vi "conversionConfigU8.vi"(1 "Config":T1={"action"=enum."PIV", "nb_periodes"=0, "t_periode"=1, "nb_pulse_prechauffe"=0, "nb_skip_frame_PIV"=0, "nb_skip_frame_LAT"=0, "t_FL1_start"=0, "t_FL1_stop"=0, "t_QS1_start"=0, "t_QS1_stop"=0, "t_FL2_start"=0, "t_FL2_stop"=0, "t_QS2_start"=0, "t_QS2_stop"=0, "t_LAT_start"=0, "t_LAT_stop"=0, "t_FRAME1_start"=0, "t_FRAME1_stop"=0, "t_FRAME2_start"=0, "t_FRAME2_stop"=0}) -> (0 "TrameConsigne":string)   [LabVIEW 2023]
uses:
  configFPGA.ctl
  convU16[U8].vi
  convU32[U8].vi
panel:
  out "size(s)":i32
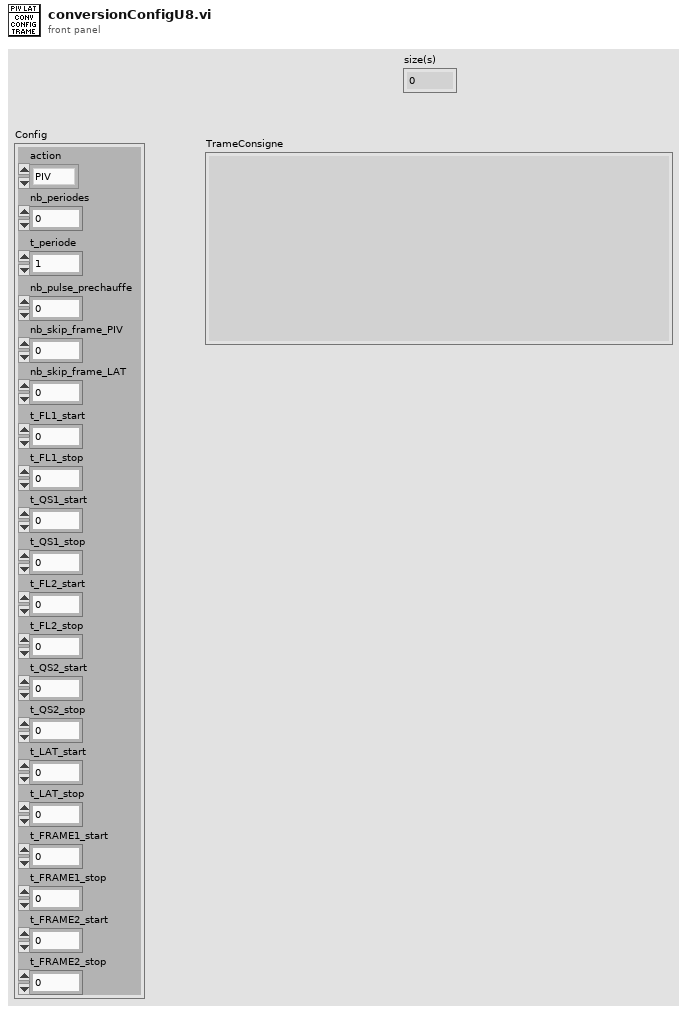
[diagram p1: front panel]
types:
  T1 = typedef "configFPGA.ctl" = cluster{"action":enum8{"PIV", "PIV + LAT", "LAT", "STOP"}, "nb_periodes":u16, "t_periode":u32, "nb_pulse_prechauffe":u8, "nb_skip_frame_PIV":u8, "nb_skip_frame_LAT":u8, "t_FL1_start":u32, "t_FL1_stop":u32, "t_QS1_start":u32, "t_QS1_stop":u32, "t_FL2_start":u32, "t_FL2_stop":u32, "t_QS2_start":u32, "t_QS2_stop":u32, "t_LAT_start":u32, "t_LAT_stop":u32, "t_FRAME1_start":u32, "t_FRAME1_stop":u32, "t_FRAME2_start":u32, "t_FRAME2_stop":u32}
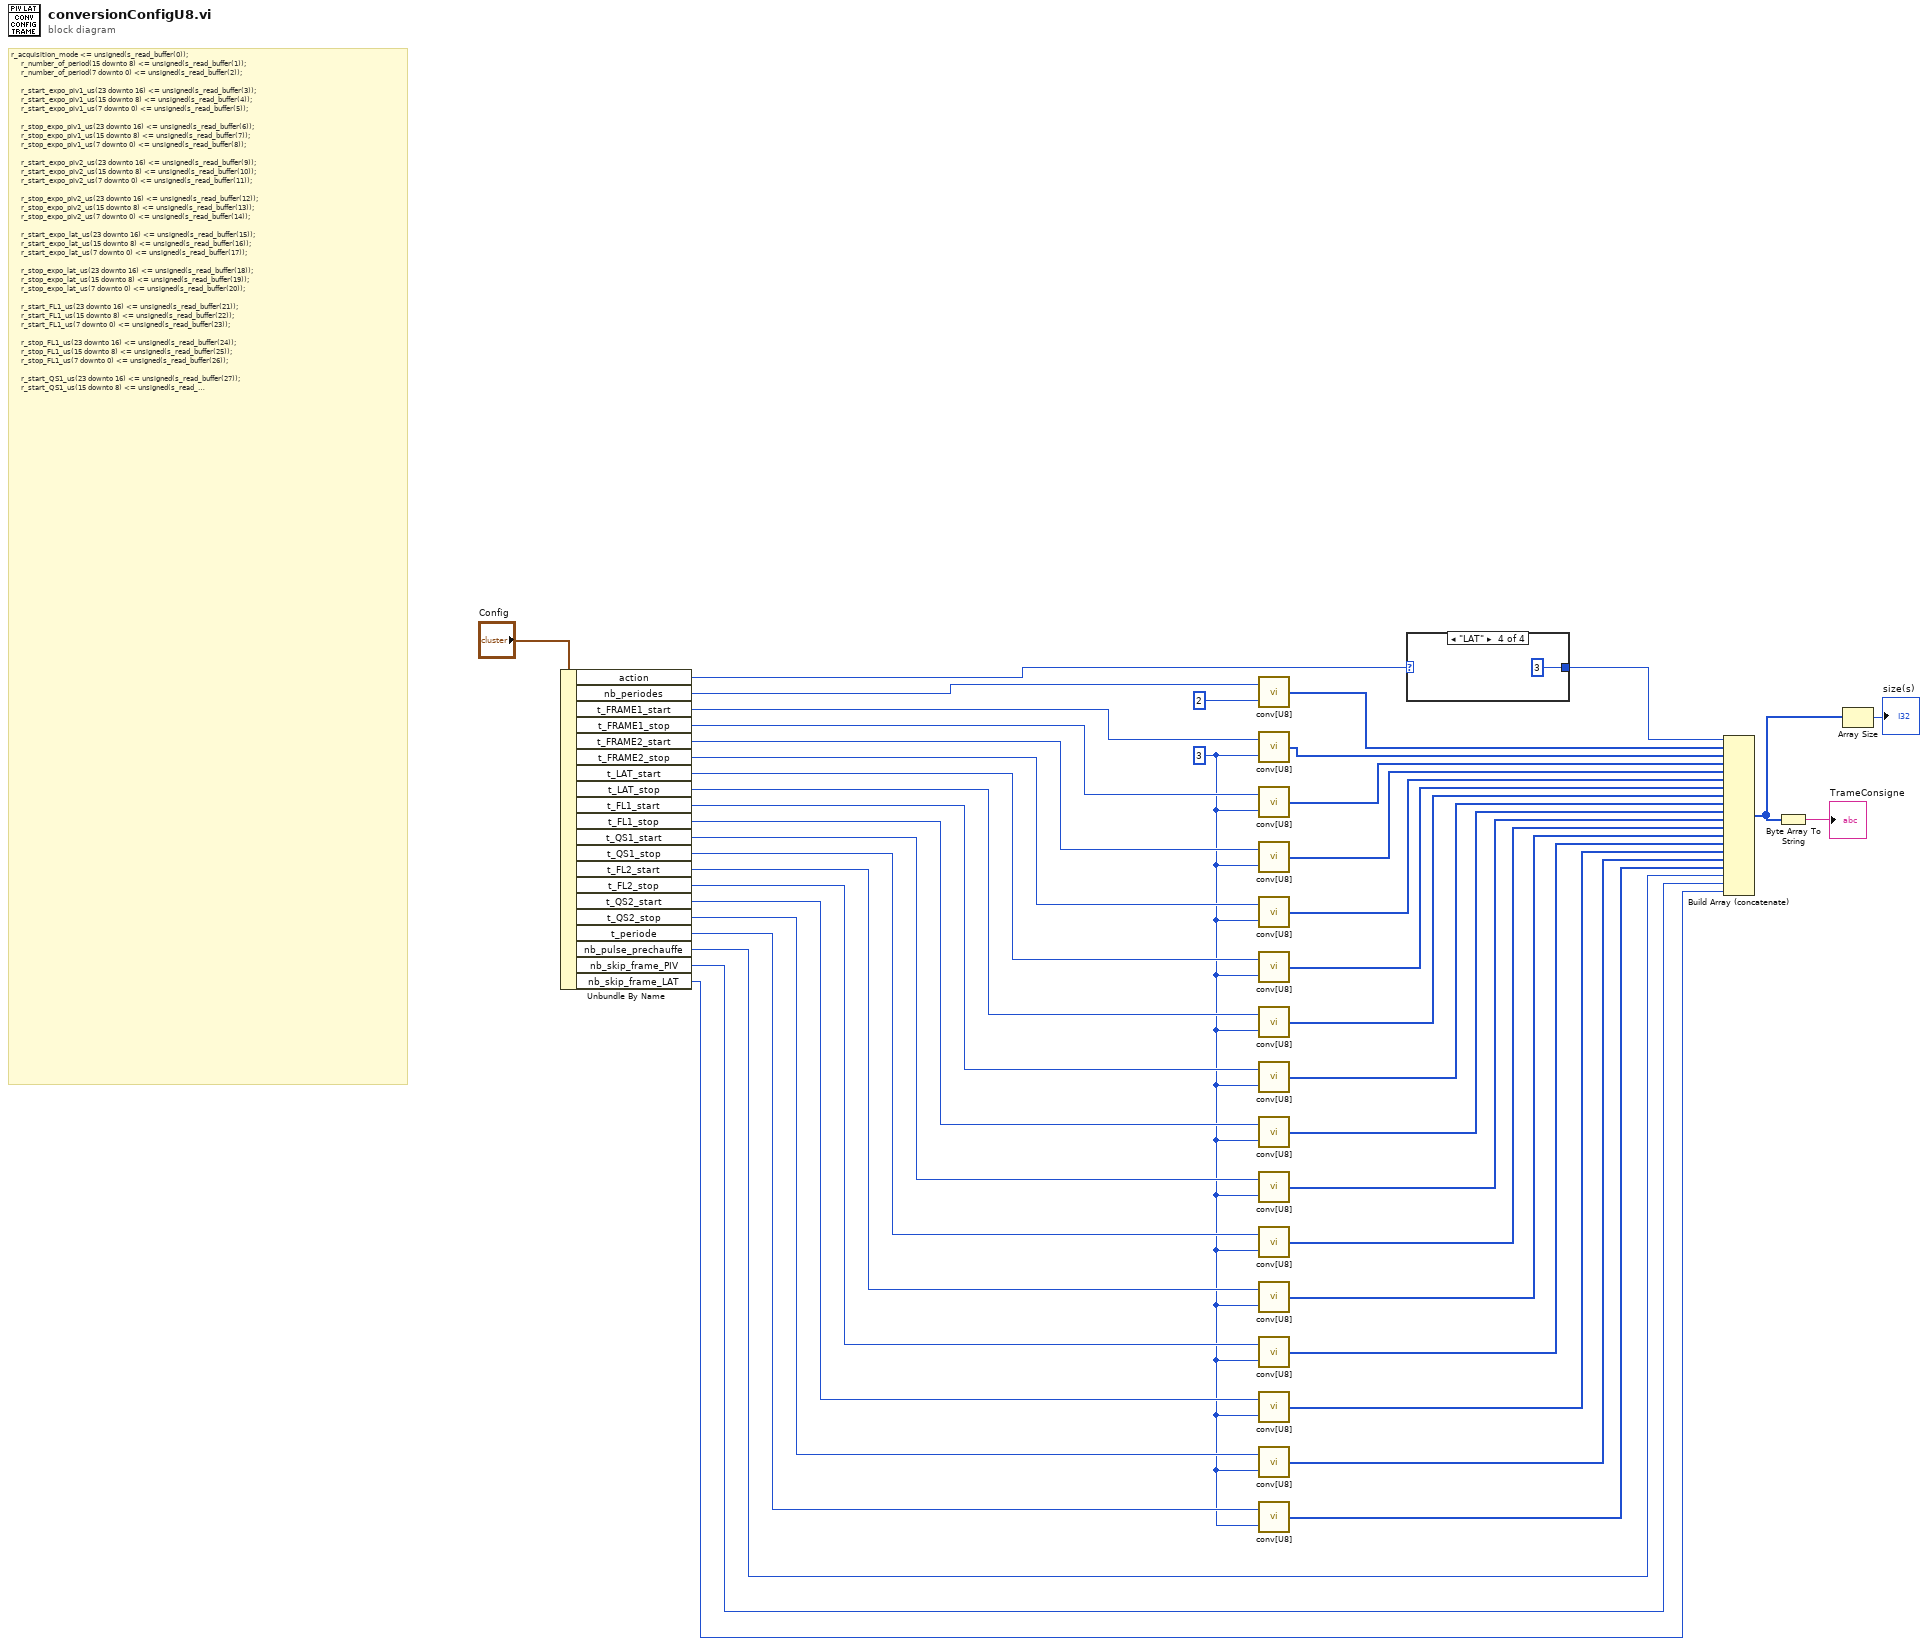
[diagram p0: block diagram]
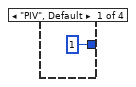
[diagram p2: hidden frame]
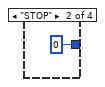
[diagram p3: hidden frame]
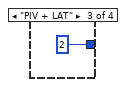
[diagram p4: hidden frame]
diagram:
  w17 = 3 ("dimension size")
  # "r_acquisition_mode <= unsigned(s_read_buffer(0));\n     r_number_of_period(15 downto 8) <= unsigned(s_read_buffer(1));\n\t\t\t\t\tr_number_of_period(7 downto 0) <= unsigned(s_read_buffer(2));\n\t\t\t\t\t\n\t\t\t\t\tr_start_expo_piv1_us(23 downto 16) <= unsigned(s_read_buffer(3));\n\t\t\t\t\tr_start_expo_piv1_us(15 downto 8) <= unsigned(s_read_buffer(4));\n\t\t\t\t\tr_start_expo_piv1_us(7 downto 0) <= unsigned(s_read_buffer(5));\n\t\t\t\t\t\n\t\t\t\t\tr_stop_expo_piv1_us(23 downto 16) <= unsigned(s_read_buffer(6));\n\t\t\t\t\tr_stop_expo_piv1_us(15 downto 8) <= unsigned(s_read_buffer(7));\n\t\t\t\t\tr_stop_expo_piv1_us(7 downto 0) <= unsigned(s_read_buffer(8));\n\t\t\t\t\t\n\t\t\t\t\tr_start_expo_piv2_us(23 downto 16) <= unsigned(s_read_buffer(9));\n\t\t\t\t\tr_start_expo_piv2_us(15 downto 8) <= unsigned(s_read_buffer(10));\n\t\t\t\t\tr_start_expo_piv2_us(7 downto 0) <= unsigned(s_read_buffer(11));\n\t\t\t\t\t\n\t\t\t\t\tr_stop_expo_piv2_us(23 downto 16) <= unsigned(s_read_buffer(12));\n\t\t\t\t\tr_stop_expo_piv2_us(15 downto 8) <= unsigned(s_read_buffer(13));\n\t\t\t\t\tr_stop_expo_piv2_us(7 downto 0) <= unsigned(s_read_buffer(14));\n\t\t\t\t\t\n\t\t\t\t\tr_start_expo_lat_us(23 downto 16) <= unsigned(s_read_buffer(15));\n\t\t\t\t\tr_start_expo_lat_us(15 downto 8) <= unsigned(s_read_buffer(16));\n\t\t\t\t\tr_start_expo_lat_us(7 downto 0) <= unsigned(s_read_buffer(17));\n\t\t\t\t\t\n\t\t\t\t\tr_stop_expo_lat_us(23 downto 16) <= unsigned(s_read_buffer(18));\n\t\t\t\t\tr_stop_expo_lat_us(15 downto 8) <= unsigned(s_read_buffer(19));\n\t\t\t\t\tr_stop_expo_lat_us(7 downto 0) <= unsigned(s_read_buffer(20));\n\t\t\t\t\t\n\t\t\t\t\tr_start_FL1_us(23 downto 16) <= unsigned(s_read_buffer(21));\n\t\t\t\t\tr_start_FL1_us(15 downto 8) <= unsigned(s_read_buffer(22));\n\t\t\t\t\tr_start_FL1_us(7 downto 0) <= unsigned(s_read_buffer(23));\n\t\t\t\t\t\n\t\t\t\t\tr_stop_FL1_us(23 downto 16) <= unsigned(s_read_buffer(24));\n\t\t\t\t\tr_stop_FL1_us(15 downto 8) <= unsigned(s_read_buffer(25));\n\t\t\t\t\tr_stop_FL1_us(7 downto 0) <= unsigned(s_read_buffer(26));\n\t\t\t\t\t\n\t\t\t\t\tr_start_QS1_us(23 downto 16) <= unsigned(s_read_buffer(27));\n\t\t\t\t\tr_start_QS1_us(15 downto 8) <= unsigned(s_read_buffer(28));\n\t\t\t\t\tr_start_QS1_us(7 downto 0) <= unsigned(s_read_buffer(29));\n\t\t\t\t\t\n\t\t\t\t\tr_stop_QS1_us(23 downto 16) <= unsigned(s_read_buffer(30));\n\t\t\t\t\tr_stop_QS1_us(15 downto 8) <= unsigned(s_read_buffer(31));\n\t\t\t\t\tr_stop_QS1_us(7 downto 0) <= unsigned(s_read_buffer(32));\n\t\t\t\t\t\n\t\t\t\t\tr_start_FL2_us(23 downto 16) <= unsigned(s_read_buffer(33));\n\t\t\t\t\tr_start_FL2_us(15 downto 8) <= unsigned(s_read_buffer(34));\n\t\t\t\t\tr_start_FL2_us(7 downto 0) <= unsigned(s_read_buffer(35));\n\t\t\t\t\t\n\t\t\t\t\tr_stop_FL2_us(23 downto 16) <= unsigned(s_read_buffer(36));\n\t\t\t\t\tr_stop_FL2_us(15 downto 8) <= unsigned(s_read_buffer(37));\n\t\t\t\t\tr_stop_FL2_us(7 downto 0) <= unsigned(s_read_buffer(38));\n\t\t\t\t\t\n\t\t\t\t\tr_start_QS2_us(23 downto 16) <= unsigned(s_read_buffer(39));\n\t\t\t\t\tr_start_QS2_us(15 downto 8) <= unsigned(s_read_buffer(40));\n\t\t\t\t\tr_start_QS2_us(7 downto 0) <= unsigned(s_read_buffer(41));\n\t\t\t\t\t\n\t\t\t\t\tr_stop_QS2_us(23 downto 16) <= unsigned(s_read_buffer(42));\n\t\t\t\t\tr_stop_QS2_us(15 downto 8) <= unsigned(s_read_buffer(43));\n\t\t\t\t\tr_stop_QS2_us(7 downto 0) <= unsigned(s_read_buffer(44));\n\t\t\t\t\t\n\t\t\t\t\tw_i_period_us(23 downto 16) <= unsigned(s_read_buffer(45));\n\t\t\t\t\tw_i_period_us(15 downto 8) <= unsigned(s_read_buffer(46));\n\t\t\t\t\tw_i_period_us(7 downto 0) <= unsigned(s_read_buffer(47));\n\t\t\t\t\t\n\t\t\t\t\tr_number_pulse_heat_laser(7 downto 0) <= unsigned(s_read_buffer(48));\n\t\t\t\t\t\n\t\t\t\t\tr_PIV_skip_frames(7 downto 0) <= unsigned(s_read_buffer(49));\n\t\t\t\t\t\n\t\t\t\t\tr_LAT_skip_frames(7 downto 0) <= unsigned(s_read_buffer(50));"
  n1 = Unbundle By Name("Config") -> ("action"=w42:enum8{"PIV", "PIV + LAT", "LAT", "STOP"}, "nb_periodes"=w34:u16, "t_FRAME1_start"=w33:u32, "t_FRAME1_stop"=w32:u32, "t_FRAME2_start"=w19:u32, "t_FRAME2_stop"=w20:u32, "t_LAT_start"=w21:u32, "t_LAT_stop"=w22:u32, "t_FL1_start"=w23:u32, "t_FL1_stop"=w24:u32, "t_QS1_start"=w25:u32, "t_QS1_stop"=w26:u32, "t_FL2_start"=w27:u32, "t_FL2_stop"=w28:u32, "t_QS2_start"=w29:u32, "t_QS2_stop"=w30:u32, "t_periode"=w18:u32, "nb_pulse_prechauffe"=w41:u8, "nb_skip_frame_PIV"=w40:u8, "nb_skip_frame_LAT"=w39:u8)
  n2 = call-poly "conv[U8].vi"("dimension size"=2, "DATA IN"=w34) -> ("DATA OUT"=w1:u8[])
  n3 = call-poly "conv[U8].vi"("dimension size"=w17, "DATA IN"=w33) -> ("DATA OUT"=w2:u8[])
  n4 = call-poly "conv[U8].vi"("dimension size"=w17, "DATA IN"=w32) -> ("DATA OUT"=w3:u8[])
  n5 = call-poly "conv[U8].vi"("dimension size"=w17, "DATA IN"=w19) -> ("DATA OUT"=w4:u8[])
  n6 = call-poly "conv[U8].vi"("dimension size"=w17, "DATA IN"=w20) -> ("DATA OUT"=w5:u8[])
  n7 = call-poly "conv[U8].vi"("dimension size"=w17, "DATA IN"=w21) -> ("DATA OUT"=w6:u8[])
  n8 = call-poly "conv[U8].vi"("dimension size"=w17, "DATA IN"=w22) -> ("DATA OUT"=w7:u8[])
  n9 = call-poly "conv[U8].vi"("dimension size"=w17, "DATA IN"=w23) -> ("DATA OUT"=w8:u8[])
  n10 = call-poly "conv[U8].vi"("dimension size"=w17, "DATA IN"=w24) -> ("DATA OUT"=w9:u8[])
  n11 = call-poly "conv[U8].vi"("dimension size"=w17, "DATA IN"=w25) -> ("DATA OUT"=w10:u8[])
  n12 = call-poly "conv[U8].vi"("dimension size"=w17, "DATA IN"=w26) -> ("DATA OUT"=w11:u8[])
  n13 = call-poly "conv[U8].vi"("dimension size"=w17, "DATA IN"=w27) -> ("DATA OUT"=w12:u8[])
  n14 = call-poly "conv[U8].vi"("dimension size"=w17, "DATA IN"=w28) -> ("DATA OUT"=w13:u8[])
  n15 = call-poly "conv[U8].vi"("dimension size"=w17, "DATA IN"=w29) -> ("DATA OUT"=w14:u8[])
  n16 = call-poly "conv[U8].vi"("dimension size"=w17, "DATA IN"=w30) -> ("DATA OUT"=w15:u8[])
  n17 = call-poly "conv[U8].vi"("dimension size"=w17, "DATA IN"=w18) -> ("DATA OUT"=w16:u8[])
  n18 = case shown="\"LAT\"" w42 {
    tunnel: [u8 1 u8 0 u8 2 u8 3] -> w35
    frame "PIV", Default {
    }
    frame "STOP" {
    }
    frame "PIV + LAT" {
    }
    frame "LAT" {
    }
  }
  n19 = Build Array (concatenate)(w35, w1, w2, w3, w4, w5, w6, w7, w8, w9, w10, w11, w12, w13, w14, w15, w16, w41, w40, w39) -> (w37:u8[])
  n20 = Byte Array To String(unsigned byte array=w37) -> (string=→"TrameConsigne":string)
  n21 = Array Size(array=w37) -> (size(s)=→"size(s)":i32)
